vi "nonlinearity.vi"() -> ()   [LabVIEW 2018]
uses:
  <vilib>/Utility/file.llb/Read Delimited Spreadsheet (DBL).vi
panel:
  out "Prepared by \nthe project":string
  out "Number \nof Cycles":i32
  out "Slope":dbl
  out "% Max \nnon-linearity \nvalue":dbl
  out "Max \nnon-linearity \nvalue":dbl
  out "x2":dbl
  out "x1":dbl
  out "y2":dbl
  out "y1":dbl
  in  "Enter The Number \nof Measurements":i32
  out "N (Difference in mA)":sgl[](array[numeric])
  out "Calculated Out(mA)":sgl[](array[numeric])
  out "Measured Out (mA)":sgl[](array[numeric])
  out "In (kg)":sgl[](array[numeric])
  in  "Measurement file \nwith extension Txt":path
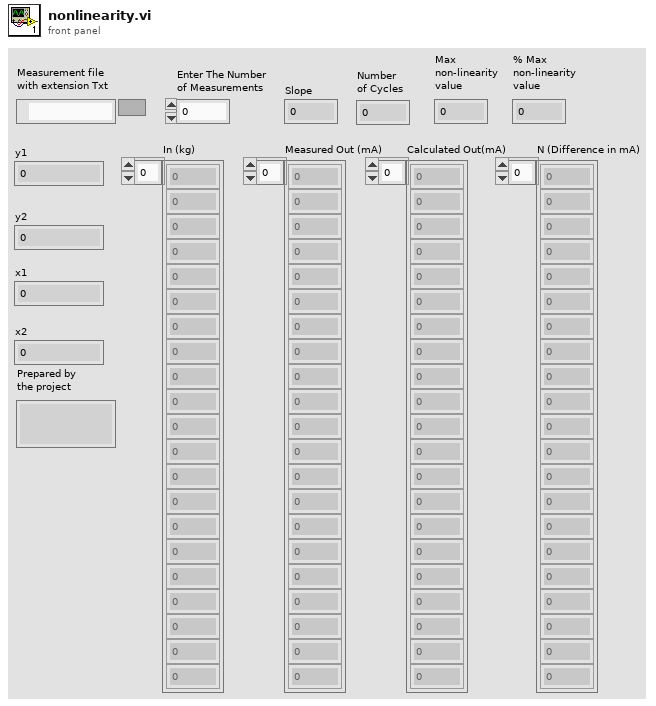
[diagram p1: front panel]
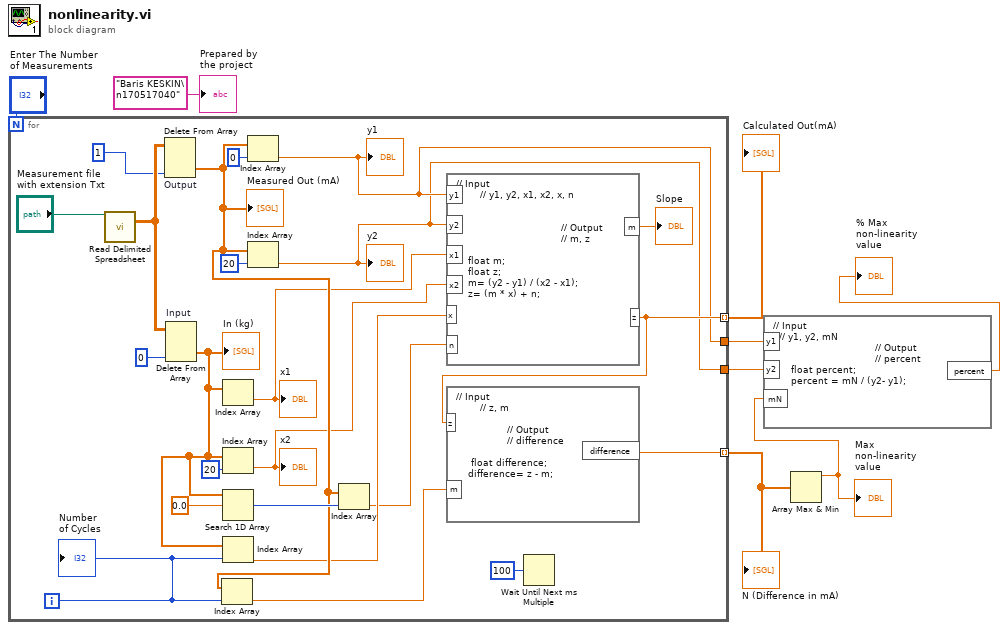
[diagram p0: block diagram]
diagram:
  n1 = for {
    N: "Enter The Number \nof Measurements" -> [_]
    tunnel: [w13] -> w7 mode=indexing
    tunnel: [w12] -> w4 mode=indexing
    tunnel: [w11] -> w6
    tunnel: [w10] -> w5
    i -> [w20]
    n2 = call-poly <vilib>:"Read Delimited Spreadsheet.vi"("file path (dialog if empty)"="Measurement file \nwith extension Txt") -> ("all rows"=w30:dbl[][])  [unwired: 9 in, 5 out]
    n3 = Delete From Array "Output"(array=w30, index (col)=1 ("disabled index (col)")) -> (deleted portion=w21:dbl[])  [unwired: 2 in, 1 out]
    "Measured Out (mA)" <- w21
    n4 = Delete From Array "Input"(array=w30, index (col)=0 ("disabled index (col)")) -> (deleted portion=w22:dbl[])  [unwired: 2 in, 1 out]
    "In (kg)" <- w22
    n5 = Index Array(array=w21, index=w20) -> (element=w14:dbl)
    n6 = Index Array(array=w22) -> (element=w19:dbl)  [unwired: 1 in]
    "x1" <- w19
    n7 = Index Array(array=w22, index=20) -> (element=w18:dbl)
    "x2" <- w18
    n8 = Search 1D Array(1D array=w22, element=0.0) -> (index of element=w23:i32)  [unwired: 1 in]
    n9 = Index Array(array=w22, index=w20) -> (element=w17:dbl)
    n10 = Index Array(array=w21, index=0) -> (element=w11:dbl)
    "y1" <- w11
    n11 = Index Array(array=w21, index=20) -> (element=w10:dbl)
    "y2" <- w10
    n12 = Index Array(array=w21, index=w23) -> (element=w16:dbl)
    n13 = formula code="// Input\n        // y1, y2, x1, x2, x, n\n    \n\n                                   // Output\n                                   // m, z\n\n    float m;\n    float z;\n    m= (y2 - y1) / (x2 - x1);\n    z= (m * x) + n;"("y1"=w11, "y2"=w10, "x1"=w19, "x2"=w18, "x"=w17, "n"=w16) -> ("m"=→"Slope":dbl, "z"=w13:dbl)
    n14 = formula code="// Input\n        // z, m\n\n                 // Output\n                 // difference\n   \n     float difference;\n    difference= z - m;"("z"=w13, "m"=w14) -> ("difference"=w12:dbl)
    n15 = Wait Until Next ms Multiple(millisecond multiple=u32 100) -> ()  [unwired: 1 out]
    "Number \nof Cycles" <- w20
  }
  "Calculated Out(mA)" <- w7
  "N (Difference in mA)" <- w4
  n16 = Array Max & Min(array=w4) -> (max value=w3:dbl)  [unwired: 3 out]
  "Max \nnon-linearity \nvalue" <- w3
  n17 = formula code="// Input \n  // y1, y2, mN\n                                  // Output\n                                  // percent\n      float percent;\n      percent = mN / (y2- y1);"("y1"=w6, "y2"=w5, "mN"=w3) -> ("percent"=→"% Max \nnon-linearity \nvalue":dbl)
  "Prepared by \nthe project" <- "Baris KESKIN\n170517040"
